vi "GetTimeStr.vi"(3 "UTC? (F)":bool) -> (1 "UTC string":string)   [LabVIEW 2011]
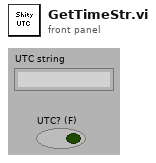
[diagram p1: front panel]
types:
  T1 = typedef "LVDateTimeRec.ctl" = cluster{"fractional second":dbl, "second":i32, "minute":i32, "hour":i32, "day of month":i32, "month":i32, "year":i32, "day of week":i32, "day of year":i32, "DST":i32}
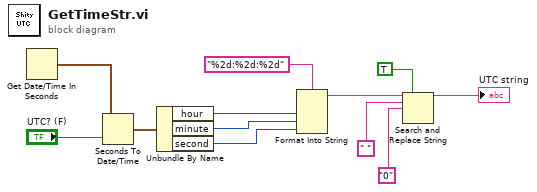
[diagram p0: block diagram]
diagram:
  n1 = Get Date/Time In Seconds() -> (seconds since 1Jan1904=w12:timestamp)
  n2 = Seconds To Date/Time(time stamp (now)=w12, to UTC (F)="UTC? (F)") -> (date time rec=w10:T1)
  n3 = Unbundle By Name(w10) -> ("hour"=w9:i32, "minute"=w8:i32, "second"=w7:i32)
  n4 = Format Into String(format string="%2d:%2d:%2d", w9, w8, w7) -> (resulting string=w5:string)  [unwired: 2 in, 1 out]
  n5 = Search and Replace String(replace all?=TRUE ("replace all? (F)"), input string=w5, search string=" ", replace string="0" ("search string")) -> (result string=→"UTC string":string)  [unwired: 4 in, 3 out]
